vi "update_zc_info3.vi"(4 "ywxinxi":string, 6 "didian":string, 8 "number":string, 9 "syren":string, 11 "status":string) -> (1 "data_str":string)   [LabVIEW 2017, in "Lib_code.lvlib"]
uses:
  Lib_code.lvlib
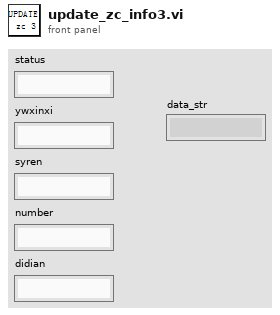
[diagram p1: front panel]
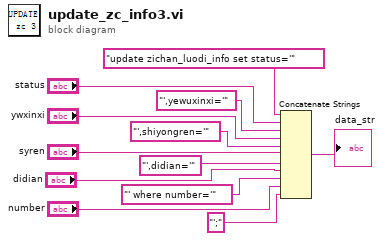
[diagram p0: block diagram]
diagram:
  n1 = Concatenate Strings("update zichan_luodi_info set status='" ("Command Text"), "status", "',yewuxinxi='" ("字符串"), "ywxinxi", "',shiyongren='" ("字符串"), "syren", "',didian='" ("字符串"), "didian", "' where number='" ("字符串"), "number", "';" ("字符串")) -> (→"data_str":string)
